vi "E443X_ESG_VSG_Configure_Amplitude.vi"(0 "VISA Resource Name":refnum<visa-resource-name>, 1 "Ampl Ref Set (0.00)":dbl format="%.2f", 2 "Ampl Ref (F:OFF)":bool, 3 "Ampl Offset (0.00)":dbl format="%.2f", 5 "Amplitude (-135.00)":dbl=-135.0 format="%.2f", 7 "Unit (0:dBm)":T1(ring), 9 "Atten Hold (F:OFF)":bool, 11 "error in (no error)":errorcluster {"code" format="%.0x"}) -> (4 "VISA Resource Name Out":refnum<visa-resource-name>, 15 "error out":errorcluster {"code" format="%.0x"})   [LabVIEW 2015]
doc: "This VI is used to set the modulation controls and the parameters associated with the signal generator's RF output amplitude."
panel:
  # "ON"
  # "OFF"
  # "ON"
  # "OFF"
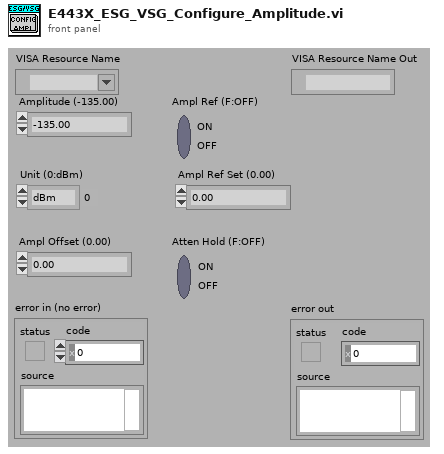
[diagram p1: front panel]
types:
  T1 = enum16{"dBm", "dBuV", "dBuVemf", "mV", "uV", "mVemf", "uVemf"}
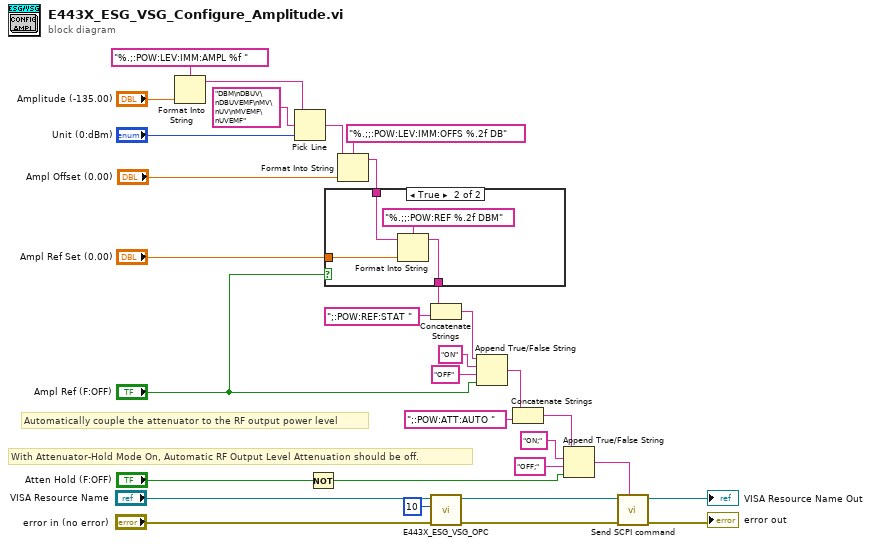
[diagram p0: block diagram]
diagram:
  # "With Attenuator-Hold Mode On, Automatic RF Output Level Attenuation should be off."
  # "Automatically couple the attenuator to the RF output power level"
  n1 = Format Into String(format string="%.;:POW:LEV:IMM:AMPL %f ", "Amplitude (-135.00)") -> (resulting string=w25:string)  [unwired: 2 in, 1 out]
  n2 = Pick Line(string ("")=w25, multi-line string="DBM\nDBUV\nDBUVEMF\nMV\nUV\nMVEMF\nUVEMF", line index="Unit (0:dBm)") -> (output string=w28:string)
  n3 = Not(x="Atten Hold (F:OFF)") -> (.not. x?=w6:bool)
  n4 = Format Into String(format string="%.;;:POW:LEV:IMM:OFFS %.2f DB", initial string=w28, "Ampl Offset (0.00)") -> (resulting string=w12:string)  [unwired: 1 in, 1 out]
  n5 = case shown="True" "Ampl Ref (F:OFF)" {
    tunnel: w12 -> [w32 w35]
    tunnel: "Ampl Ref Set (0.00)" -> [_ w34]
    tunnel: [w32 w33] -> w10
    frame False {
    }
    frame True {
      n6 = Format Into String(format string="%.;;:POW:REF %.2f DBM", initial string=w35, w34) -> (resulting string=w33:string)  [unwired: 1 in, 1 out]
    }
  }
  n7 = Concatenate Strings(w10, ";:POW:REF:STAT ") -> (w8:string)
  n8 = call "E443X_ESG_VSG_OPC.vi"("error in (no error)"="error in (no error)", "Wait (1000ms)"=u32 10, "VISA resource name"="VISA Resource Name") -> ("error out"=w4:errorcluster, "VISA resource name out"=w2:refnum<visa-resource-name>)  [unwired: 7 in]
  n9 = Append True/False String(1:"Ampl Ref (F:OFF)", 2:"OFF" ("false string"), 3:"ON" ("true string"), 4:w8) -> (0:w18:string)
  n10 = Concatenate Strings(w18, ";:POW:ATT:AUTO ") -> (w17:string)
  n11 = Append True/False String(1:w6, 2:"OFF;" ("false string"), 3:"ON;" ("true string"), 4:w17) -> (0:w5:string)
  n12 = call "Send SCPI command.vi"("Send SCPI Command"=w5, "error in (no error)"=w4, "VISA resource name"=w2) -> ("error out"=→"error out":errorcluster, "VISA resource name out"=→"VISA Resource Name Out":refnum<visa-resource-name>)  [unwired: 7 in]
